vi "Add Enqueuer.vi"(9 "Nested Enqueuer":refnum<class "Message Enqueuer.lvclass">, 10 "Ident":string, 11 "Panel Actor Template in":refnum<class "Network Management UI.lvclass">) -> (3 "Panel Actor Template out":refnum<class "Network Management UI.lvclass">)   [LabVIEW 2024, in "Network Management UI.lvlib" / "Network Management UI.lvclass"]
uses:
  Network Management UI.lvclass
  Network Management UI.lvclass/Network Management UI.ctl
  <vilib>/ActorFramework/Message Enqueuer/Message Enqueuer.lvclass
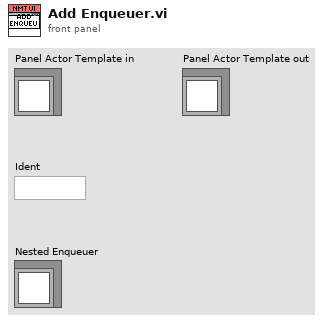
[diagram p1: front panel]
types:
  T1 = map{string, refnum<class "Message Enqueuer.lvclass">}
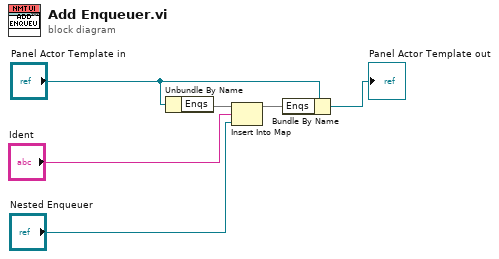
[diagram p0: block diagram]
diagram:
  n1 = Unbundle By Name("Panel Actor Template in") -> ("Enqs"=w6:T1)
  n2 = Insert Into Map(map in=w6, key="Ident", value="Nested Enqueuer") -> (map out=w3:T1)  [unwired: 2 out]
  n3 = Bundle By Name(cluster="Panel Actor Template in", "Enqs"=w3) -> (→"Panel Actor Template out":refnum<class "Network Management UI.lvclass">)
